vi "OpenSF.vi"(1 "port number":u16) -> (0 "error out":errorcluster, 2 "read buffer 5":string, 3 "connection ID":refnum<k5>)   [LabVIEW 2011]
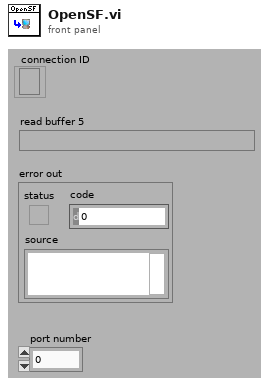
[diagram p1: front panel]
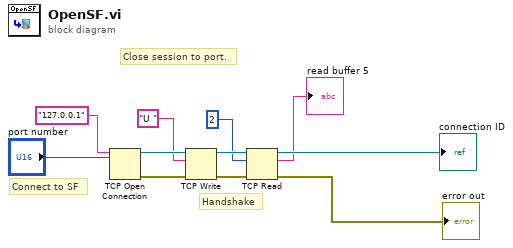
[diagram p0: block diagram]
diagram:
  # "Handshake"
  # "Connect to SF"
  # "Close session to port."
  n1 = TCP Open Connection(address="127.0.0.1", remote port or service name="port number") -> (connection ID=w6:refnum<k5>, error out=w5:errorcluster)  [unwired: 3 in]
  n2 = TCP Write(connection ID=w6, data in="U ", error in (no error)=w5) -> (connection ID out=w7:refnum<k5>, error out=w8:errorcluster)  [unwired: 1 in, 1 out]
  n3 = TCP Read(connection ID=w7, bytes to read=2, error in (no error)=w8) -> (connection ID out=→"connection ID":refnum<k5>, data out=→"read buffer 5":string, error out=→"error out":errorcluster)  [unwired: 2 in]
